vi "test sensors assignemt.vi"() -> ()   [LabVIEW 2020]
uses:
  <vilib>/Utility/file.llb/Read Delimited Spreadsheet (DBL).vi
  <vilib>/addons/control/pid/pid.llb/PID (DBL).vi
  <vilib>/ptbypt/NI_PtbyPt.lvlib
  <vilib>/addons/control/pid/NI_PID_pid.lvlib
panel:
  out "Waveform Chart 3":dbl(graph)
  out "Waveform Chart 2":dbl(graph)
  in  "output range":cluster{"output high":dbl, "output low":dbl}={"output high"=100.0, "output low"=-100.0} {"output low" format="%.2f"; "output high" format="%.2f"}
  in  "PID gains":T1={"proportional gain (Kc)"=1.0, "integral time (Ti, min)"=0.01, "derivative time (Td, min)"=0.0} {"derivative time (Td, min)" format="%.3f"; "integral time (Ti, min)" format="%.3f"; "proportional gain (Kc)" format="%.3f"}
  in  "file path (dialog if empty)":path
  out "Mass (g)":dbl
  out "Force (N)":dbl
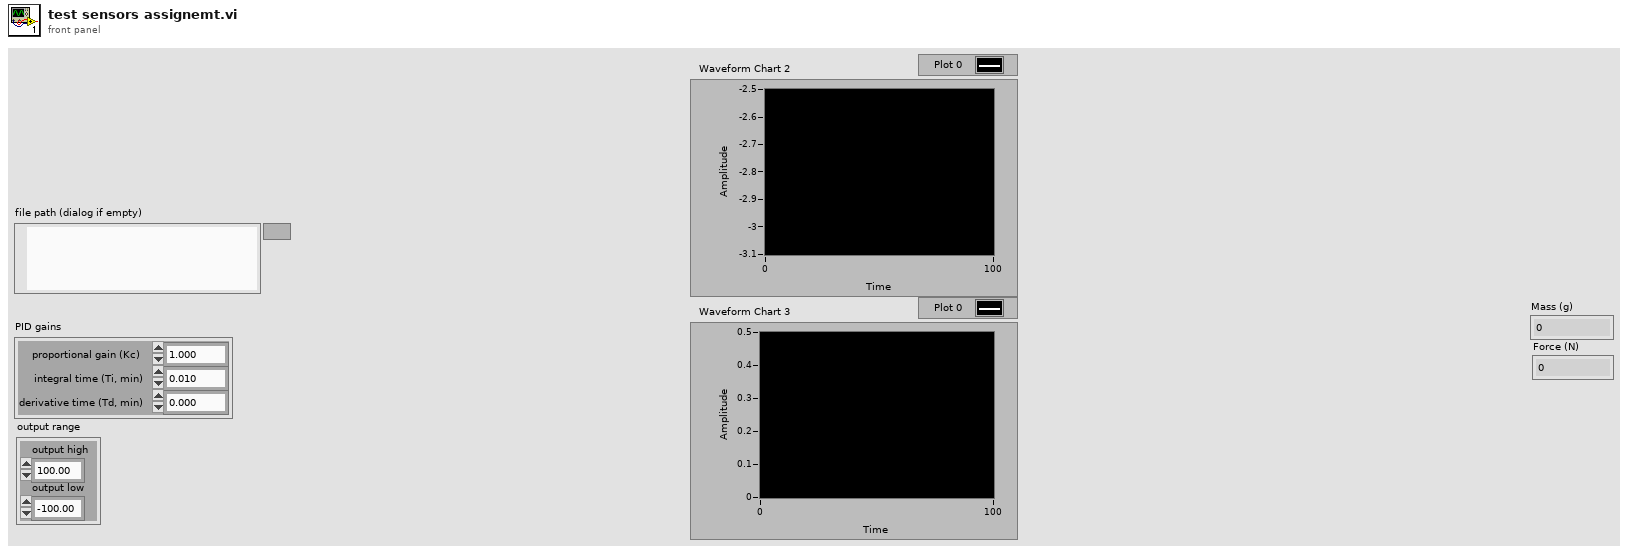
[diagram p1: front panel]
types:
  T1 = cluster{"proportional gain (Kc)":dbl, "integral time (Ti, min)":dbl, "derivative time (Td, min)":dbl}
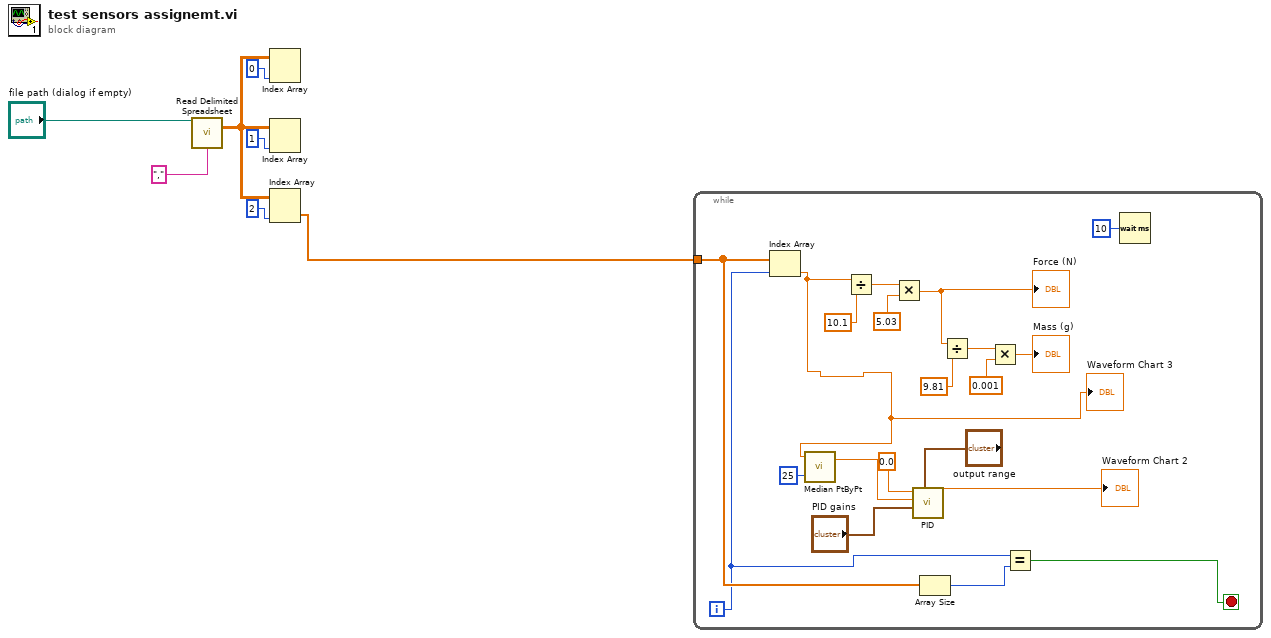
[diagram p0: block diagram]
diagram:
  n1 = call-poly <vilib>:"Read Delimited Spreadsheet.vi"("file path (dialog if empty)"="file path (dialog if empty)", "delimiter (\\t)"="," ("delimiter (\\t)")) -> ("all rows"=w7:dbl[][])  [unwired: 8 in, 5 out]
  n2 = Index Array(array=w7, index (col)=0 ("disabled index (col)")) -> ()  [unwired: 1 in, 1 out]
  n3 = Index Array(array=w7, index (col)=1 ("disabled index (col)")) -> ()  [unwired: 1 in, 1 out]
  n4 = Index Array(array=w7, index (col)=2 ("disabled index (col)")) -> (element=w1:dbl[])  [unwired: 1 in]
  n5 = while {
    tunnel: w1 -> [w17]
    i -> [w11]
    stop <- w16 stop-if-true
    n6 = Index Array(array=w17, index=w11) -> (element=w8:dbl)
    "Waveform Chart 3" <- w8
    n7 = call <vilib>:"Median PtByPt.vi"("sample length"=25, "x"=w8) -> ("median"=w14:dbl)  [unwired: 2 in, 1 out]
    n8 = Divide(x=w8, y=10.1) -> (x/y=w24:dbl)
    n9 = Multiply(x=w24, y=5.03) -> (x*y=w27:dbl)
    "Force (N)" <- w27
    n10 = call-poly <vilib>:"PID.vi"("output range"="output range", "PID gains"="PID gains", "process variable"=w14, "setpoint"=0.0) -> ("output"=→"Waveform Chart 2":dbl)  [unwired: 6 in, 1 out]
    n11 = Array Size(array=w17) -> (size(s)=w18:i32)
    n12 = Divide(x=w27, y=9.81) -> (x/y=w25:dbl)
    n13 = Multiply(x=w25, y=0.001) -> (x*y=→"Mass (g)":dbl)
    n14 = Equal?(x=w11, y=w18) -> (x = y?=w16:bool)
    n15 = Wait (ms)(milliseconds to wait=u32 10) -> ()  [unwired: 1 out]
  }
